vi "New Frame.vi"(8 "error in (no error)":errorcluster, 10 "Frame Number\n(starts with 1)":i32, 11 "Particle Counter in":refnum<class "Particle Counter.lvclass">) -> (0 "error out":errorcluster, 3 "Particle Counter out":refnum<class "Particle Counter.lvclass">)   [LabVIEW 2023, in "Particle Counter.lvlib" / "Particle Counter.lvclass"]
uses:
  Particle Counter.lvclass
  Particle Counter.lvclass/Particle Counter.ctl
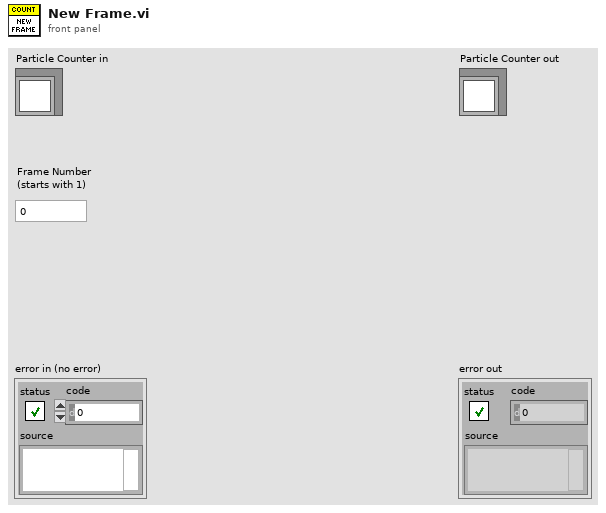
[diagram p1: front panel]
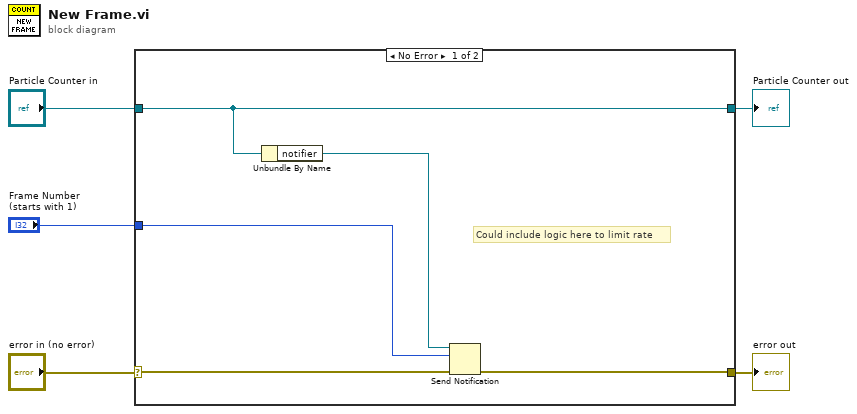
[diagram p0: block diagram]
diagram:
  n1 = case shown="No Error" "error in (no error)" {
    selector: "error in (no error)" -> [w9 w12]
    tunnel: [w8 w12] -> w4
    tunnel: [w10 w11] -> w2
    tunnel: "Particle Counter in" -> [w10 w11]
    tunnel: "Frame Number\n(starts with 1)" -> [w6 _]
    frame No Error {
      # "Could include logic here to limit rate"
      n2 = Unbundle By Name(w10) -> ("notifier"=w7:refnum<notifier>)
      n3 = Send Notification(notification=w6, notifier=w7, error in (no error)=w9) -> (error out=w8:errorcluster)  [unwired: 1 out]
    }
    frame Error {
    }
  }
  "error out" <- w4
  "Particle Counter out" <- w2
